vi "Scale joystick data.vi"(1 "Factor X":dbl format="%.2f", 2 "Factor Y":dbl format="%.2f", 3 "XPos":i32, 4 "YPos":i32, 6 "XPos Center":i32, 7 "YPos Center":i32, 8 "Dead band X":i32, 9 "Dead band Y":i32) -> (14 "XPos scaled":i32, 15 "YPos scaled":i32)   [LabVIEW 2026]
doc: "Sub-VI for operation with a joystick connected to the game port of the host computer. Scales joystick position. Use output value from Calculate joystick scaling.vi for Factor *. Dead band * is the maximum scaled position value that does not result in any motion."
panel:
  # "Scales joystick position. Use output value from \"Calculate joystick scaling.vi\" for \"Factor *\".\nDead band is maximum size of scaled position value that doesn't result in any motion."
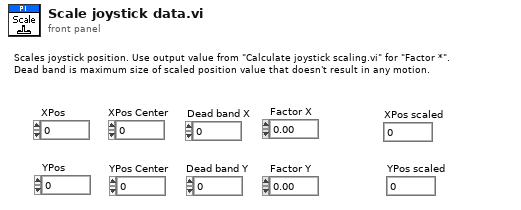
[diagram p1: front panel]
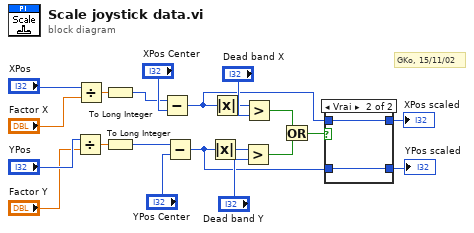
[diagram p0: block diagram]
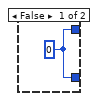
[diagram p2: hidden frame]
diagram:
  # "GKo, 15/11/02"
  n1 = Divide(x="YPos", y="Factor Y") -> (x/y=w17:dbl)
  n2 = Divide(x="XPos", y="Factor X") -> (x/y=w19:dbl)
  n3 = To Long Integer(number=w19) -> (32bit integer=w11:i32)
  n4 = To Long Integer(number=w17) -> (32bit integer=w10:i32)
  n5 = Subtract(x=w11, y="XPos Center") -> (x-y=w8:i32)
  n6 = Subtract(x=w10, y="YPos Center") -> (x-y=w7:i32)
  n7 = Absolute Value(x=w7) -> (abs(x)=w1:i32)
  n8 = Absolute Value(x=w8) -> (abs(x)=w2:i32)
  n9 = Greater?(x=w1, y="Dead band Y") -> (0:w12:bool)
  n10 = Greater?(x=w2, y="Dead band X") -> (0:w13:bool)
  n11 = Or(x=w13, y=w12) -> (x .or. y?=w9:bool)
  n12 = case shown="Vrai" w9 {
    tunnel: [w22 w24] -> w6
    tunnel: w8 -> [_ w24]
    tunnel: w7 -> [_ w23]
    tunnel: [w22 w23] -> w5
    frame False {
      w22 = 0
    }
    frame True {
    }
  }
  "XPos scaled" <- w6
  "YPos scaled" <- w5
